vi "Header Value.vi"(8 "error in (no error)":errorcluster, 9 "Default (Empty)":string, 10 "Header":string, 11 "Request in":refnum<class "Request.lvclass">) -> (0 "error out":errorcluster, 1 "Exists":bool, 2 "Value":string, 3 "Request out":refnum<class "Request.lvclass">)   [LabVIEW 2020, in "HTTP Utils.lvlib" / "Request.lvclass"]
uses:
  Request.lvclass
  Request.lvclass/Request.ctl
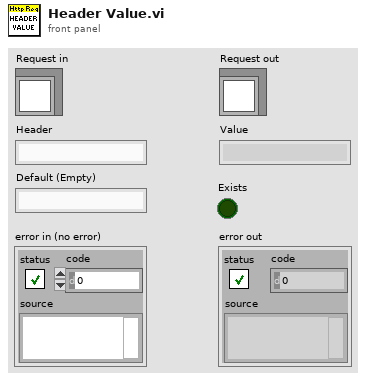
[diagram p1: front panel]
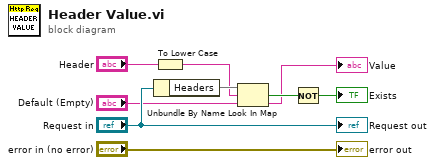
[diagram p0: block diagram]
diagram:
  n1 = Unbundle By Name("Request in") -> ("Headers"=w7:map{string, string})
  n2 = To Lower Case(string="Header") -> (all lower case string=w4:string)
  n3 = Look In Map(map=w7, key=w4, default value="Default (Empty)") -> (key not found?=w3:bool, value=→"Value":string)
  n4 = Not(x=w3) -> (.not. x?=→"Exists":bool)
  "error out" <- "error in (no error)"
  "Request out" <- "Request in"
